vi "Set Sequencer Msg Priority.vi"(8 "error in (no error)":errorcluster, 10 "Message Priority":T1, 11 "Flex Msg in":refnum<class "Flex Msg.lvclass">) -> (0 "error out":errorcluster, 3 "Flex Msg out":refnum<class "Flex Msg.lvclass">)   [LabVIEW 2020, in "Sequencer.lvlib"]
doc: "Set Msg priority if part of the Sequencer Msg class hierarchy."
uses:
  Sequencer.lvlib
  PPL/HDH.Actor Framework.Core.Actor.lvlibp/1abvi3w/vi.lib/ActorFramework/Message Enqueuer/Message Priority.ctl
  PPL/HDH.Actor Framework.Core.Msg.lvlibp/Flex Msg/Flex Msg.lvclass
  Sequencer Messages/Sequencer Msg/Sequencer Msg.lvclass
  C:/Current projects/WS/PPL/HDH.Actor Framework.Core.Msg.lvlibp/Flex Msg/Flex Msg.lvclass
  Sequencer Messages/Sequencer Msg/Sequencer Msg.lvclass/Sequencer Msg.ctl
  PPL/HDH.Actor Framework.Core.Actor.lvlibp/1abvi3w/vi.lib/ActorFramework/Message Enqueuer/Message Enqueuer.lvclass
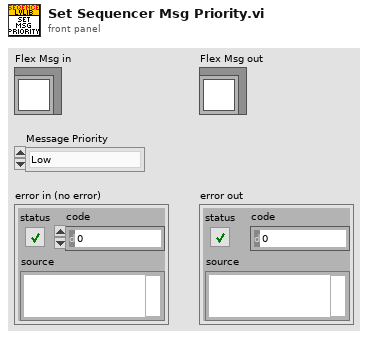
[diagram p1: front panel]
types:
  T1 = typedef "HDH.Actor Framework.Core.Actor.lvlibp/Message Enqueuer.lvclass/Message Priority.ctl" = enum16{"Low", "Normal", "High"}
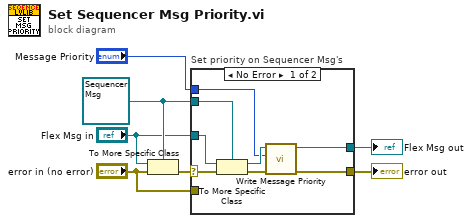
[diagram p0: block diagram]
diagram:
  w7 = refnum<class "Sequencer Msg.lvclass"> refnum ("Sequencer.lvlib:Sequencer Msg.lvclass")
  n1 = To More Specific Class(target class=w7, reference="Flex Msg in", error in="error in (no error)") -> (error out=w1:errorcluster)  [unwired: 1 out]
  n2 = case "Set priority on Sequencer Msg's" shown="No Error" w1 {
    selector: w1 -> [w15 _]
    tunnel: [w9 w17] -> w3
    tunnel: "error in (no error)" -> [_ w17]
    tunnel: [w10 w16] -> w5
    tunnel: "Flex Msg in" -> [w14 w16]
    tunnel: w7 -> [w13 _]
    tunnel: "Message Priority" -> [w8 _]
    frame No Error {
      n3 = To More Specific Class(target class=w13, reference=w14, error in=w15) -> (specific class reference=w12:refnum<class "Sequencer Msg.lvclass">, error out=w11:errorcluster)
      n4 = call "Write Message Priority.vi"("error in (no error)"=w11, "Priority"=w8, "Sequencer Msg in"=w12) -> ("error out"=w9:errorcluster, "Sequencer Msg out"=w10:refnum<class "Sequencer Msg.lvclass">)  [unwired: 7 in]
    }
    frame Error {
    }
  }
  "Flex Msg out" <- w5
  "error out" <- w3
